vi "CORE Command.vi"(0 "Serial Devices in":refnum<class "Serial Devices.lvclass">, 1 "Device":string, 5 "Command":string(combo), 7 "Chanel":string, 9 "Param":string, 11 "error in (no error)":errorcluster) -> (4 "Serial Devices out":refnum<class "Serial Devices.lvclass">, 6 "Command":string, 10 "Expected":string, 15 "error out":errorcluster)   [LabVIEW 2019, in "Serial Devices.lvlib" / "Serial Devices.lvclass"]
uses:
  Serial Devices.lvclass
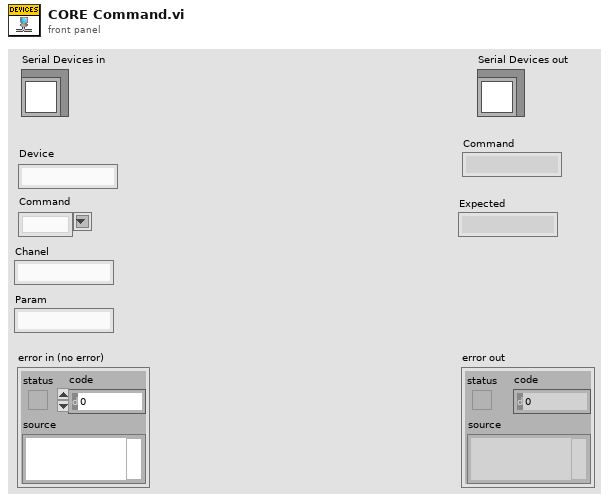
[diagram p1: front panel]
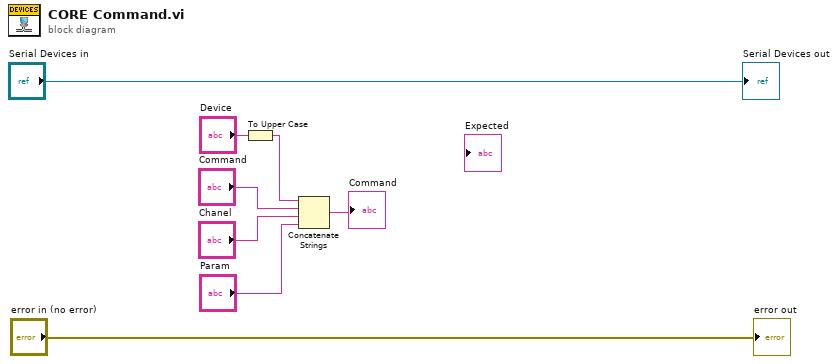
[diagram p0: block diagram]
diagram:
  n1 = To Upper Case(1:"Device") -> (0:w5:string)
  n2 = Concatenate Strings(w5, "Command", "Chanel", "Param") -> (→"Command":string)
  "error out" <- "error in (no error)"
  "Serial Devices out" <- "Serial Devices in"
